vi "DataFmt.vi"(8 "error in (no error)":errorcluster, 10 "Data Format (F:ASCII)":bool, 11 "VISA resource name":refnum<visa-resource-name>) -> (0 "error out":errorcluster, 3 "VISA resource name out":refnum<visa-resource-name>)   [LabVIEW 2015, in "Agilent 428X Series.lvlib"]
doc: "This VI is to format the data output format of the instrument.\n\nModel 4284 only."
uses:
  Agilent 428X Series.lvlib
panel:
  # "IEEE-64"
  # "ASCII"
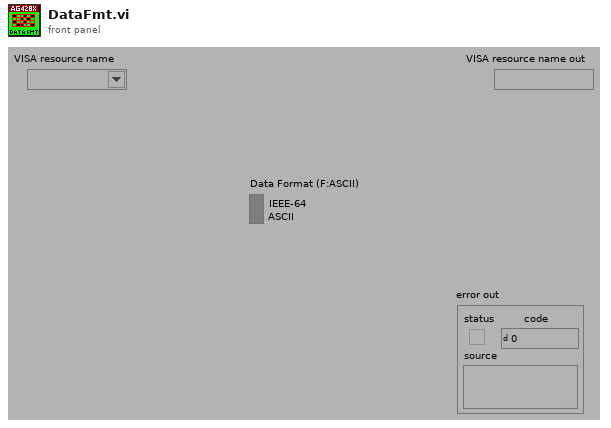
[diagram p1: front panel]
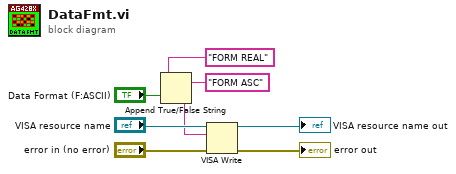
[diagram p0: block diagram]
diagram:
  n1 = Append True/False String(1:"Data Format (F:ASCII)", 2:"FORM ASC" ("false string"), 3:"FORM REAL" ("true string")) -> (0:w1:string)  [unwired: 1 in]
  n2 = VISA Write(VISA resource name="VISA resource name", write buffer=w1, error in (no error)="error in (no error)") -> (VISA resource name out=→"VISA resource name out":refnum<visa-resource-name>, error out=→"error out":errorcluster)  [unwired: 1 out]
